vi "ExecEng_ExportSequenceToFile.vi"(8 "error in (no error)":errorcluster, 11 "VI Server.RefsCluster in":T1) -> (0 "error out":errorcluster, 3 "VI Server.RefsCluster out":T1)   [LabVIEW 2020]
uses:
  LabVIEW 2020 Toolkits/VI Server Toolkit/VI Server_TypeDefs/VI Server_RefsCluster.ctl
panel:
  out "SequenceFile.SAVE.Success":bool
  in  "ArbitraryFileSelector":path caption="Arbitrary File Selector"
  in  "EXIT":bool
  in  "SequenceFile.SAVE":bool
  in  "TestCaseConfiguration":i32[](listbox) caption="Test Case Configuration"
  in  "Sequence.FileNames":u16(ring) caption="Sequence File Names:"
  in  "SequenceFile.Path":path[](array[path])
  # "EXPORT SEQUENCE TO FILE"
  # "M"
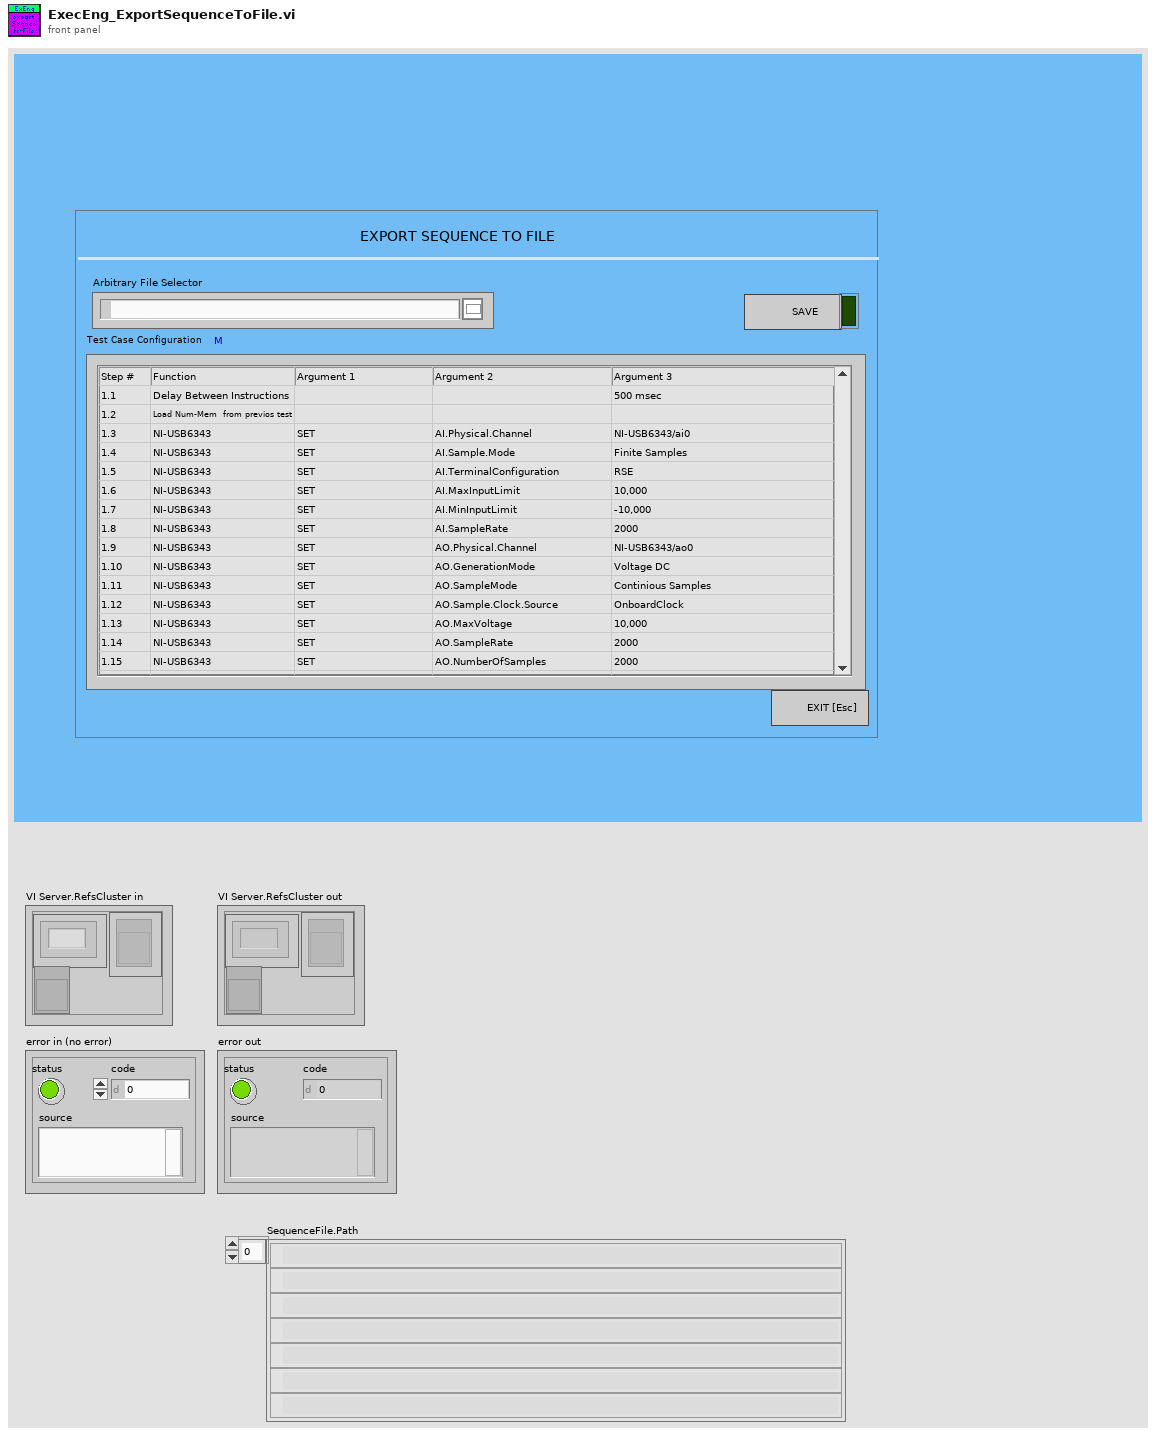
[diagram p1: front panel]
types:
  T1 = typedef "VI Server_RefsCluster.ctl" = cluster{"Labels":string[], "Refs":refnum<vi>[], "VI Ref":refnum<vi>}
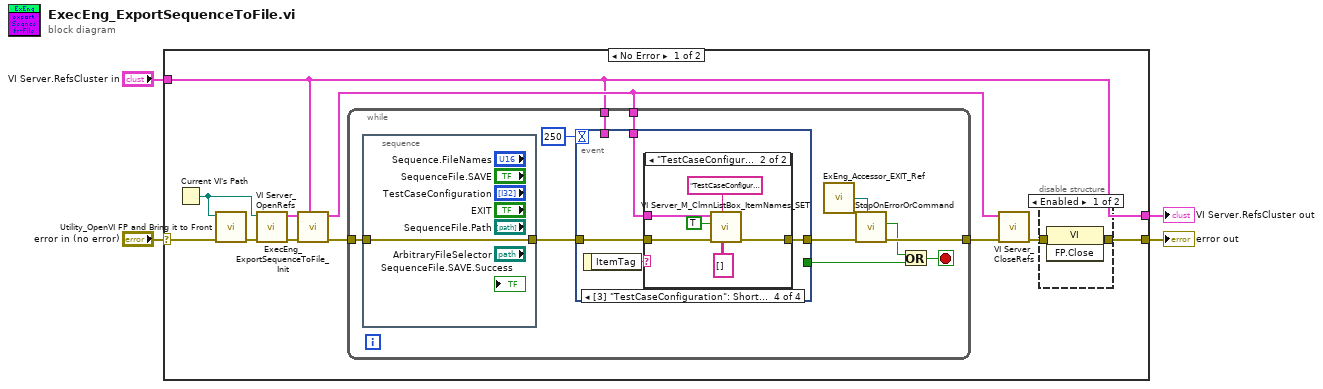
[diagram p0: block diagram]
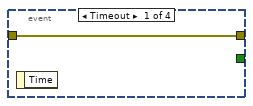
[diagram p3: hidden frame]
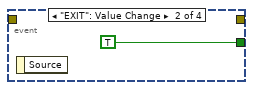
[diagram p4: hidden frame]
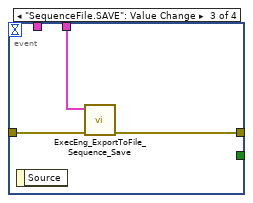
[diagram p5: hidden frame]
diagram:
  n1 = case shown="No Error" "error in (no error)" {
    selector: "error in (no error)" -> [w14 w47]
    tunnel: "VI Server.RefsCluster in" -> [w5 _]
    tunnel: [w8 w47] -> w1
    tunnel: [w5 _] -> w4
    frame No Error {
      n2 = Current VI's Path() -> (path=w6:path)
      n3 = call "Utility_OpenVI FP and Bring it to Front.vi"("error in (no error)"=w14, "VI Path"=w6) -> ("error out"=w13:errorcluster)  [unwired: 9 in]
      n4 = call "VI Server_OpenRefs.vi"("error in"=w13, "VI Path"=w6) -> ("error out"=w12:errorcluster, "VI Server.RefsCluster"=w10:T1)  [unwired: 8 in]
      n5 = call "ExecEng_ExportSequenceToFile_Init.vi"("VI Server.RefsCluster.TopVI"=w5, "error in (no error)"=w12, "VI Server.RefsCluster.Local"=w10) -> ("error out"=w15:errorcluster, "VI Server.RefsCluster.DUP"=w7:T1)  [unwired: 7 in]
      n6 = while {
        tunnel: w15 -> [w29]
        tunnel: [w25] -> w11
        tunnel: w7 -> [w21]
        tunnel: w5 -> [w20]
        stop <- w22 stop-if-true
        n7 = stacked-sequence {
          tunnel: w29 -> [w30]
          tunnel: [w30] -> w19
          frame #0 {
          }
        }
        n8 = event shown="[3] \"TestCaseConfiguration\": Shortcut Menu Selection (User)" {
          selector: _ -> [_ _ _ _]
          dyn-events: _ -> [_ _ _ _]
          timeout: 250 -> [_ _ _ _]
          tunnel: [w31 _ w34 w37] -> w26
          tunnel: [_ TRUE _ _] -> w23
          tunnel: w21 -> [_ _ w33 w36]
          tunnel: w20 -> [_ _ _ _]
          tunnel: w19 -> [w31 _ w35 w38]
          event Timeout {
            n9 = event-data() -> ()  [unwired: 1 in, 1 out]
          }
          event "EXIT": Value Change {
            n10 = event-data() -> ()  [unwired: 1 in, 1 out]
          }
          event "SequenceFile.SAVE": Value Change {
            n11 = event-data() -> ()  [unwired: 1 in, 1 out]
            n12 = call "ExecEng_ExportToFile_Sequence_Save.vi"("error in (no error)"=w35, "VI Server Cluster"=w33) -> ("error out"=w34:errorcluster)  [unwired: 9 in]
          }
          event "TestCaseConfiguration": Shortcut Menu Selection (User) {
            n13 = event-data() -> ("ItemTag"=w39:string)  [unwired: 1 in]
            n14 = case shown="\"TestCaseConfiguration\"" w39 {
              tunnel: w38 -> [w40 w46]
              tunnel: [w40 w45] -> w37
              tunnel: w36 -> [_ w44]
              frame "False", Default {
              }
              frame "TestCaseConfiguration" {
                n15 = call "VI Server_M_ClmnListBox_ItemNames_SET.vi"("Item Names"=string[][] [], "Label"="TestCaseConfiguration", "error in"=w46, "SingleInstance"=TRUE, "VI Server.RefsCluster"=w44) -> ("error out"=w45:errorcluster)  [unwired: 4 in, 2 out]
              }
            }
          }
        }
        n16 = call "ExEng_Accessor_EXIT_Ref.vi"() -> ("EXIT"=w27:refnum<notifier>)  [unwired: 6 in]
        n17 = call "StopOnErrorOrCommand.vi"("STOP"=w27, "error in (no error)"=w26) -> ("error out"=w25:errorcluster, "STOP"=w24:bool)  [unwired: 8 in]
        n18 = Or(x=w24, y=w23) -> (x .or. y?=w22:bool)
      }
      n19 = call "VI Server_CloseRefs.vi"("error in"=w11, "VI Server.RefsCluster"=w7) -> ("error out"=w9:errorcluster)  [unwired: 9 in]
      n20 = disable-structure shown="Enabled" {
        disable-tunnel: w9 -> [w17 w18]
        disable-tunnel: [w16 w18] -> w8
        frame Enabled {
          n21 = invoke class="VI" method="FP.Close"(error in=w17) -> (error out=w16:errorcluster)  [unwired: 2 in, 2 out]
        }
        frame Disabled {
        }
      }
    }
    frame Error {
    }
  }
  "VI Server.RefsCluster out" <- w4
  "error out" <- w1
